vi "UsrProfiles-Generate new profile filepath.vi"(6 "New user":bool, 9 "Destination User name":string, 11 "Copied profile's filepath":path) -> (3 "Filepath of profile to be created":path)   [LabVIEW 2020]
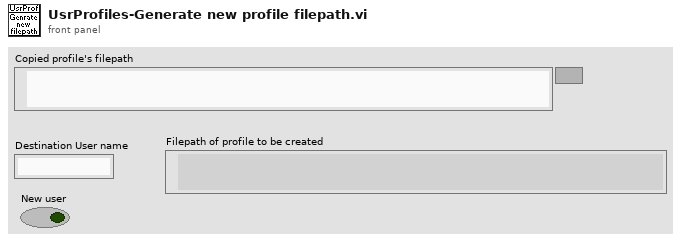
[diagram p1: front panel]
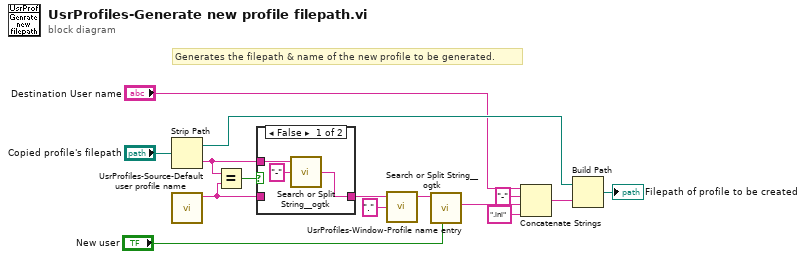
[diagram p0: block diagram]
diagram:
  # "Generates the filepath & name of the new profile to be generated."
  n1 = Strip Path(path="Copied profile's filepath") -> (stripped path=w15:path, name=w10:string)
  n2 = call "UsrProfiles-Source-Default user profile name.vi"() -> ("Default user's profile file name & extension"=w9:string)  [unwired: 11 in]
  n3 = Equal?(x=w10, y=w9) -> (x = y?=w8:bool)
  n4 = case shown="False" w8 {
    tunnel: w9 -> [_ w19]
    tunnel: w10 -> [w18 _]
    tunnel: [w17 w19] -> w3
    frame False {
      n5 = call <userlib>:"Search or Split String__ogtk.vi"("search string/char (-)"="-", "string"=w18) -> ("substring after match"=w17:string)  [unwired: 1 in, 2 out]
    }
    frame True {
    }
  }
  n6 = call <userlib>:"Search or Split String__ogtk.vi"("search string/char (-)"=".", "string"=w3) -> ("substring before match"=w4:string)  [unwired: 1 in, 2 out]
  n7 = call "UsrProfiles-Window-Profile name entry.vi"("New user"="New user", "Profile name"=w4) -> ("New profile name"=w6:string)  [unwired: 7 in, 2 out]
  n8 = Concatenate Strings("Destination User name", "-" ("string"), w6, ".ini" ("string")) -> (w13:string)
  n9 = Build Path(base path=w15, name or relative path=w13) -> (appended path=→"Filepath of profile to be created":path)
